vi "User Console View.vi"(8 "error in (no error)":errorcluster, 11 "View Model":T1) -> (0 "error out":errorcluster)   [LabVIEW 2017]
doc: "This simulated HW Console View. Contains human input."
uses:
  View Model/Controls/View Model.ctl
  Configuration/Controls/Config Model.ctl
  Configuration/Controls/Config Data.ctl
  Error Handler/Controls/Error Model.ctl
  Error Handler/Controls/Error Data.ctl
  Error Handler/Controls/Error Type.ctl
  View Model/Controls/Shared Model.ctl
  Elevator Controller/Controls/Elevator Model.ctl
  Elevator Controller/Controls/Elevator Location.ctl
  Elevator Controller/Controls/Elevator CMD Data.ctl
  Elevator Controller/Controls/Elevator Commands.ctl
  Elevator Controller/Controls/Elevator Overhead.ctl
  Elevator Controller/Controls/Elevator States.ctl
  Controls/User Console.ctl
panel:
  in  "Emergency":bool
  in  "1st Floor":bool
  in  "2nd Floor":bool
  in  "3rd Floor":bool
  in  "4th Floor":bool
  in  "Close Door":bool
  in  "Open Door":bool
  in  "Down 4":bool
  in  "Down 3":bool
  in  "Down 2":bool
  in  "Up 3":bool
  in  "Up 2":bool
  in  "Up 1":bool
  # "[Covers: UI1]"
  # "Floor Selection"
  # "Elevator Call"
  # "[Covers: UI2B]"
  # "[Covers UI2A1]"
  # "[Covers UI2A2]"
  # "[Covers UI2B2]"
  # "by controls mechanical actions"
  # "[Covers: UI2C]"
  # "[Covers: UI2D]"
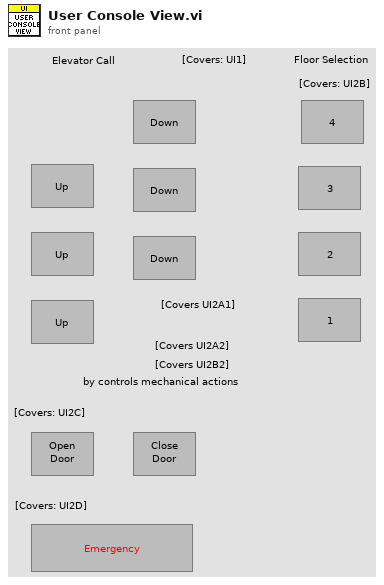
[diagram p1: front panel]
types:
  T1 = typedef "View Model.ctl" = cluster{"Config Model":T2, "Error Model":T3, "Shared Model":T4, "Elevator Model":T5}
  T2 = typedef "Config Model.ctl" = cluster{"Config Change":refnum<user-event>, "Config Data":refnum<data-value>}
  T3 = typedef "Error Model.ctl" = cluster{"Error Event":refnum<user-event>}
  T4 = typedef "Shared Model.ctl" = cluster{"Stop Event":refnum<user-event>, "Stop DVR":refnum<data-value>}
  T5 = typedef "Elevator Model.ctl" = cluster{"Motion Change":refnum<user-event>, "Direction Change":refnum<user-event>, "Door Position Change":refnum<user-event>, "Emergency Change":refnum<user-event>, "Floor Change":refnum<user-event>, "Elevator CMD":refnum<user-event>, "Controller Overhead":refnum<data-value>}
  T6 = typedef "User Console.ctl" = cluster{"Down 2":refnum<vi>, "Down 3":refnum<vi>, "Down 4":refnum<vi>, "Up 1":refnum<vi>, "Up 2":refnum<vi>, "Up 3":refnum<vi>, "1st Floor":refnum<vi>, "2nd Floor":refnum<vi>, "3rd Floor":refnum<vi>, "4th Floor":refnum<vi>, "Open Door":refnum<vi>, "Close Door":refnum<vi>, "Emergency":refnum<vi>}
  T7 = typedef "Elevator Commands.ctl" = enum16{"Go Up", "Go Down", "Go to Floor", "Emergency", "Open Doors", "Close Doors"}
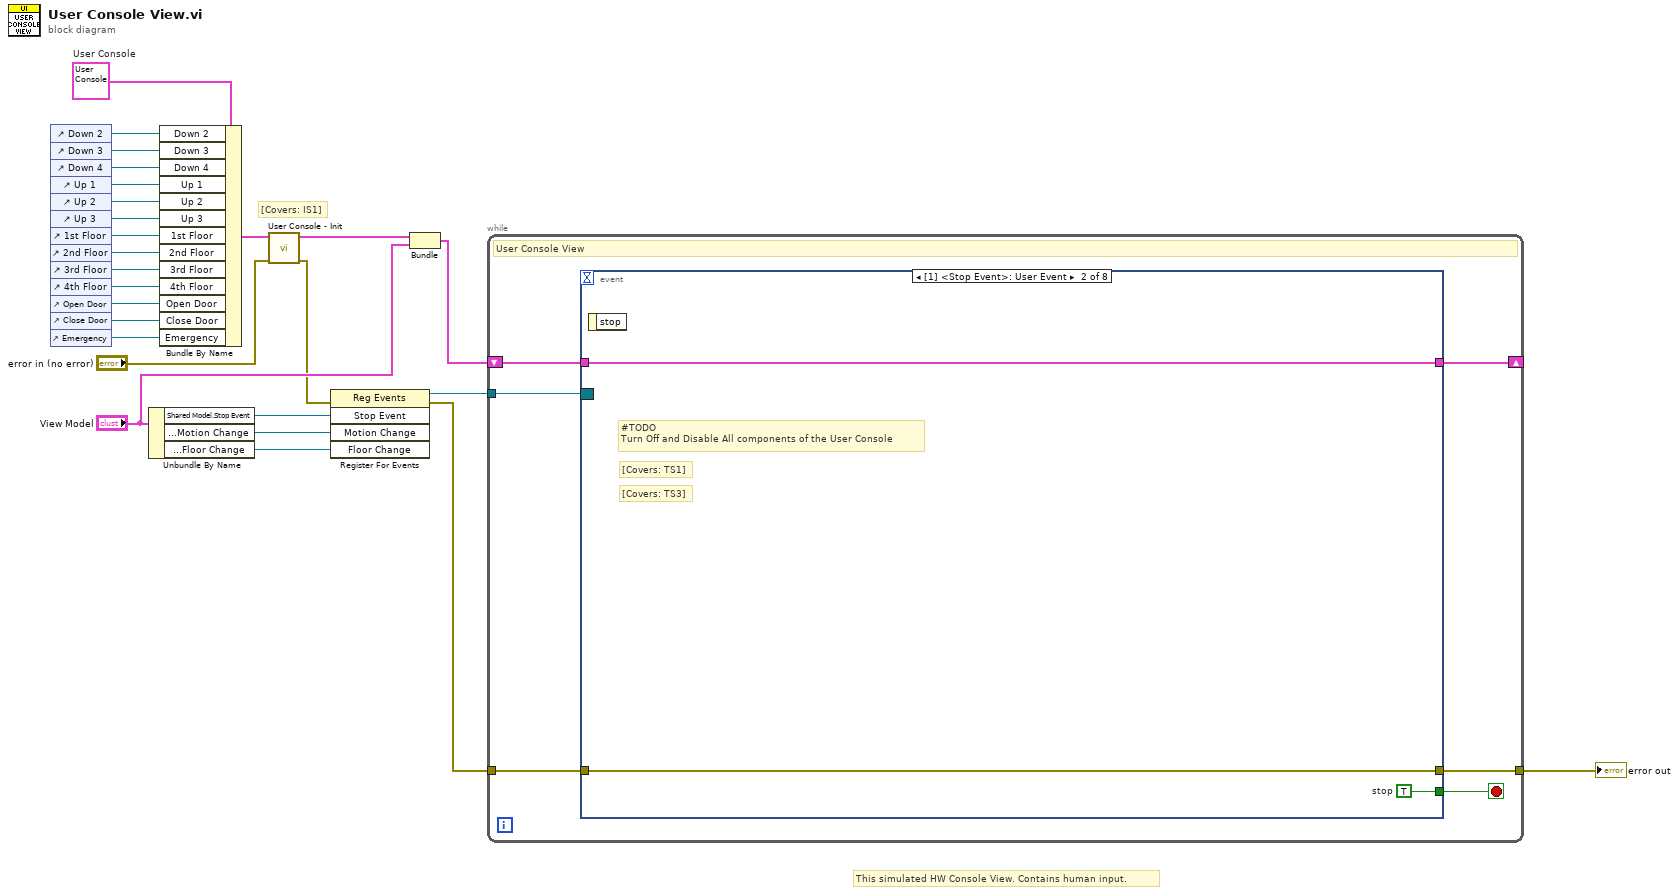
[diagram p0: block diagram]
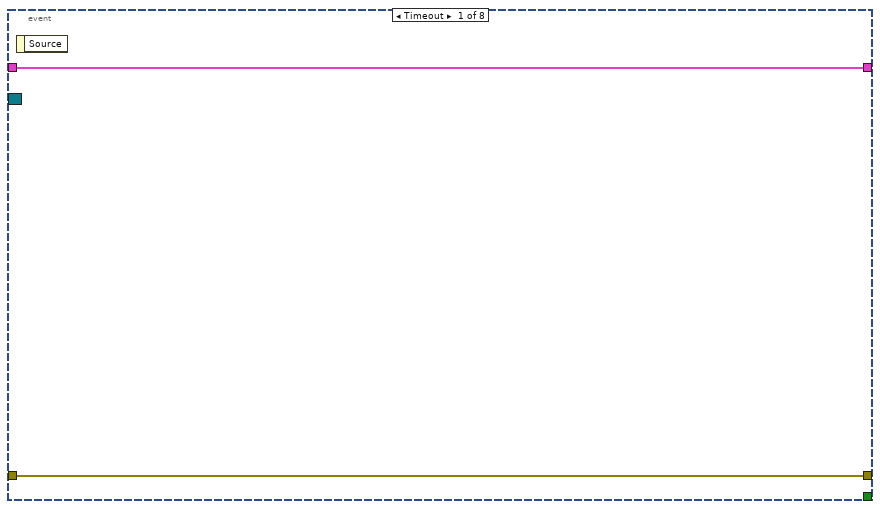
[diagram p2: hidden frame]
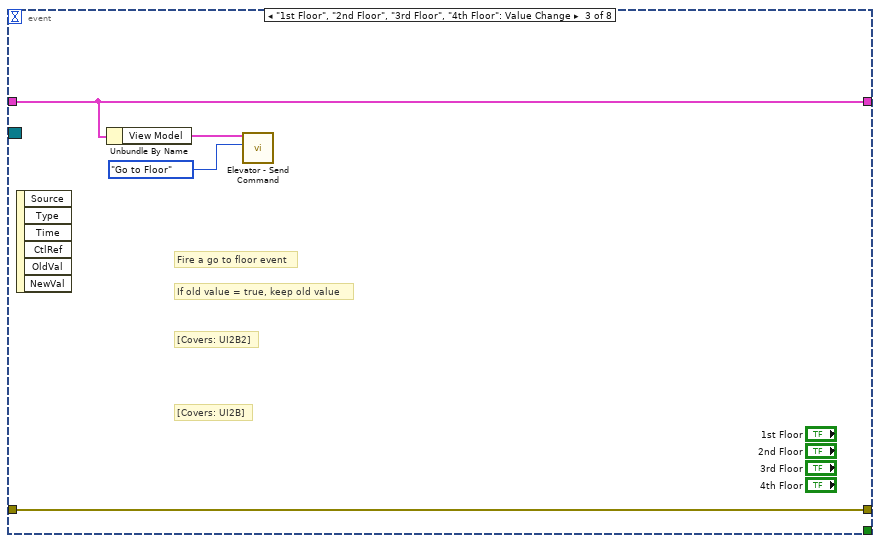
[diagram p3: hidden frame]
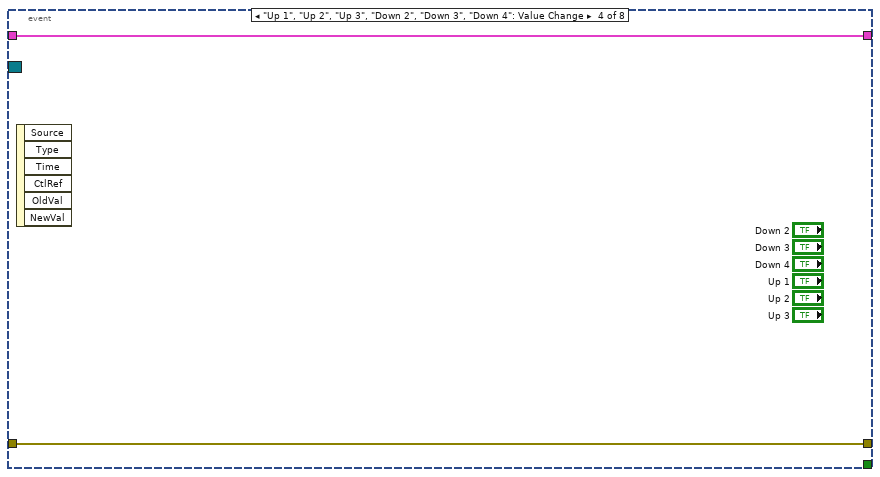
[diagram p4: hidden frame]
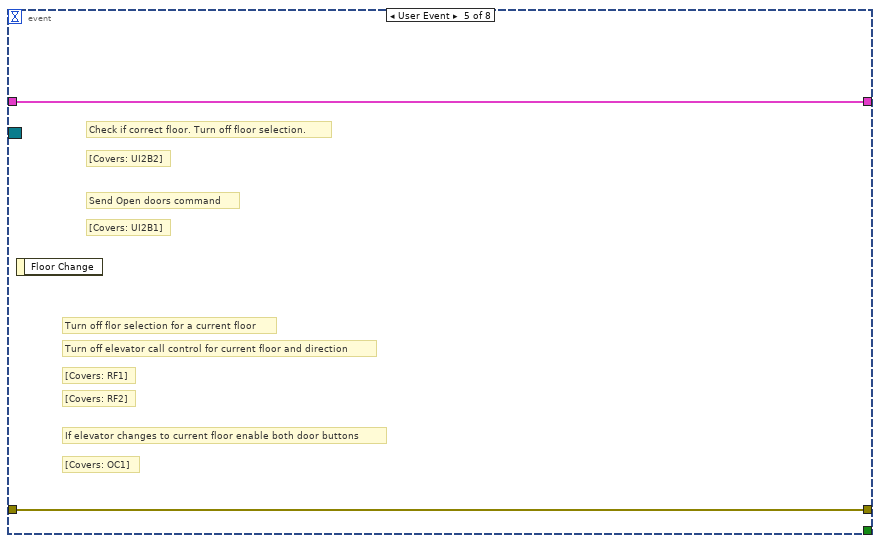
[diagram p5: hidden frame]
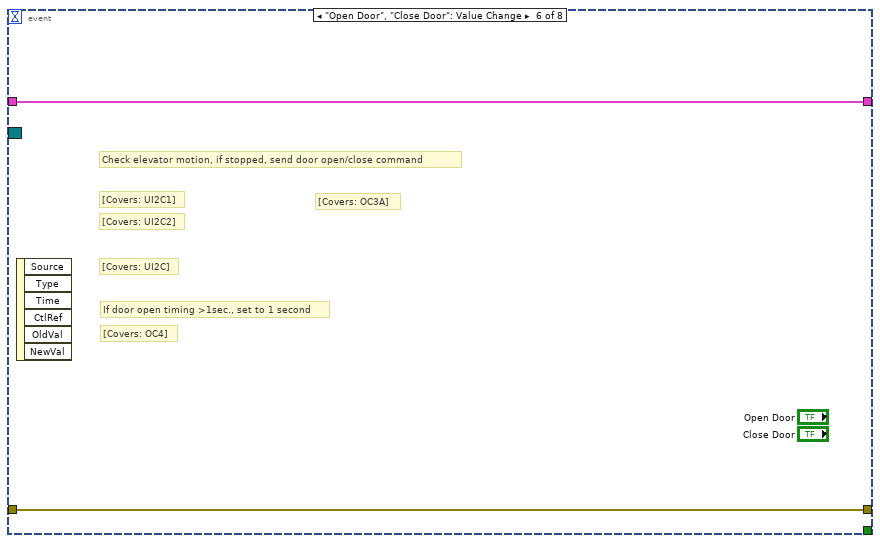
[diagram p6: hidden frame]
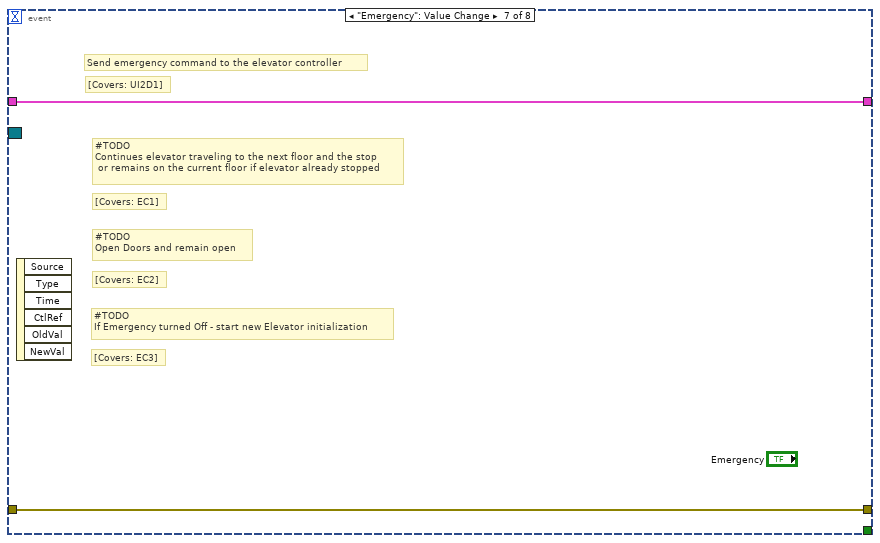
[diagram p7: hidden frame]
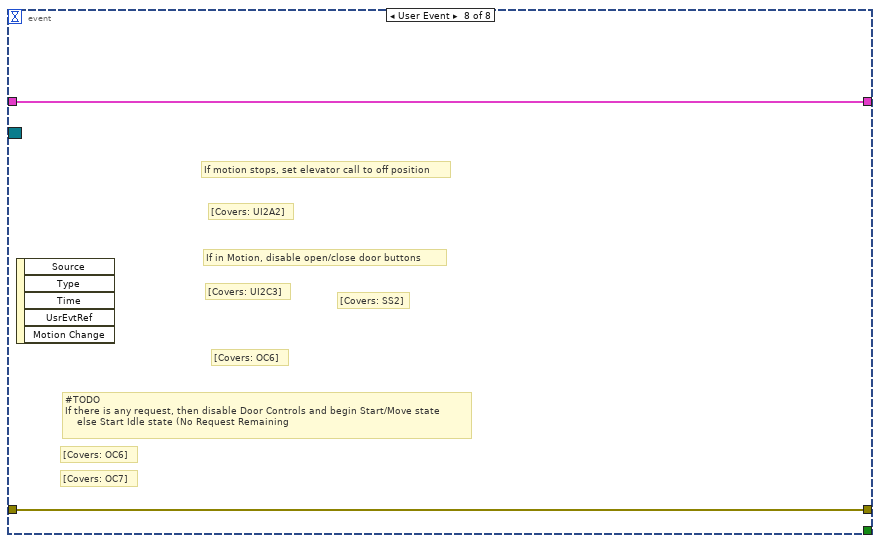
[diagram p8: hidden frame]
diagram:
  w22 = T6 {"Down 2"=refnum, "Down 3"=refnum, "Down 4"=refnum, "Up 1"=refnum, "Up 2"=refnum, "Up 3"=refnum, "1st Floor"=refnum, "2nd Floor"=refnum, "3rd Floor"=refnum, "4th Floor"=refnum, "Open Door"=refnum, "Close Door"=refnum, "Emergency"=refnum}  # User Console
  # "[Covers: IS1]"
  # "This simulated HW Console View. Contains human input."
  n1 = control-ref of="Down 2"() -> (w21:refnum<vi>)
  n2 = control-ref of="Down 3"() -> (w19:refnum<vi>)
  n3 = control-ref of="Down 4"() -> (w18:refnum<vi>)
  n4 = control-ref of="Up 1"() -> (w17:refnum<vi>)
  n5 = control-ref of="Up 2"() -> (w16:refnum<vi>)
  n6 = control-ref of="Up 3"() -> (w15:refnum<vi>)
  n7 = control-ref of="1st Floor"() -> (w14:refnum<vi>)
  n8 = control-ref of="2nd Floor"() -> (w13:refnum<vi>)
  n9 = control-ref of="3rd Floor"() -> (w12:refnum<vi>)
  n10 = control-ref of="4th Floor"() -> (w11:refnum<vi>)
  n11 = control-ref of="Open Door"() -> (w10:refnum<vi>)
  n12 = control-ref of="Close Door"() -> (w9:refnum<vi>)
  n13 = control-ref of="Emergency"() -> (w20:refnum<vi>)
  n14 = Unbundle By Name("View Model") -> ("Shared Model.Stop Event"=w26:refnum<user-event>, "Elevator Model.Motion Change"=w25:refnum<user-event>, "Elevator Model.Floor Change"=w1:refnum<user-event>)
  n15 = Bundle By Name(cluster=w22, "Down 2"=w21, "Down 3"=w19, "Down 4"=w18, "Up 1"=w17, "Up 2"=w16, "Up 3"=w15, "1st Floor"=w14, "2nd Floor"=w13, "3rd Floor"=w12, "4th Floor"=w11, "Open Door"=w10, "Close Door"=w9, "Emergency"=w20) -> (w8:T6)
  n16 = call "User Console - Init.vi"("error in (no error)"="error in (no error)", "User Console"=w8) -> ("error out"=w4:errorcluster, "User Console"=w7:T6)  [unwired: 8 in]
  n17 = register-events(error in=w4, w26, w25, w1) -> (reference out=w24:refnum<event-registration>, error out=w3:errorcluster)  [unwired: 1 in]
  n18 = Bundle("User Console"=w7, "View Model"="View Model") -> (w2:cluster{"User Console":T6, "View Model":T1})  [unwired: 1 in]
  n19 = while {
    tunnel: w24 -> [w32]
    tunnel: w3 -> [w31]
    tunnel: [w30] -> w23
    shift-right: [w27] -> _
    shift-left: w2 -> [w28]
    stop <- w29 stop-if-true
    # "User Console View"
    n20 = event shown="[1] <Stop Event>: User Event" {
      selector: w32 -> [_ _ _ _ _ _ _ _]
      dyn-events: _ -> [_ _ _ _ _ _ _ _]
      timeout: _ -> [_ _ _ _ _ _ _ _]
      tunnel: w31 -> [w34 w35 w41 w43 w45 w47 w49 w51]
      tunnel: [w34 w35 w41 w43 w45 w47 w49 w51] -> w30
      tunnel: [_ w37 _ _ _ _ _ _] -> w29
      tunnel: w28 -> [w33 w36 w40 w42 w44 w46 w48 w50]
      tunnel: [w33 w36 w40 w42 w44 w46 w48 w50] -> w27
      event Timeout {
        n21 = event-data() -> ()  [unwired: 1 in, 1 out]
      }
      event User Event {
        w37 = TRUE  # stop
        # "[Covers: TS3]"
        # "[Covers: TS1]"
        # "#TODO\nTurn Off and Disable All components of the User Console"
        n22 = event-data() -> ()  [unwired: 1 in, 1 out]
      }
      event "1st Floor", "2nd Floor", "3rd Floor", "4th Floor": Value Change {
        # "[Covers: UI2B]"
        # "[Covers: UI2B2]"
        # "If old value = true, keep old value"
        # "Fire a go to floor event"
        n23 = event-data() -> ()  [unwired: 1 in, 6 out]
        n24 = Unbundle By Name(w40) -> ("View Model"=w39:T1)
        n25 = call "Elevator - Send Command.vi"("Elevator Commands"=Elevator_Commands."Go to Floor", "View Model"=w39) -> ()  [unwired: 8 in, 2 out]
      }
      event "Up 1", "Up 2", "Up 3", "Down 2", "Down 3", "Down 4": Value Change {
        n26 = event-data() -> ()  [unwired: 1 in, 6 out]
      }
      event User Event {
        # "[Covers: UI2B1]"
        # "Send Open doors command"
        # "Check if correct floor. Turn off floor selection."
        # "[Covers: UI2B2]"
        # "[Covers: OC1]"
        # "If elevator changes to current floor enable both door buttons"
        # "[Covers: RF2]"
        # "Turn off elevator call control for current floor and direction"
        # "[Covers: RF1]"
        # "Turn off flor selection for a current floor"
        n27 = event-data() -> ()  [unwired: 1 in, 1 out]
      }
      event "Open Door", "Close Door": Value Change {
        # "[Covers: OC3A]"
        # "[Covers: UI2C]"
        # "[Covers: UI2C2]"
        # "[Covers: UI2C1]"
        # "Check elevator motion, if stopped, send door open/close command"
        # "[Covers: OC4]"
        # "If door open timing >1sec., set to 1 second"
        n28 = event-data() -> ()  [unwired: 1 in, 6 out]
      }
      event "Emergency": Value Change {
        # "[Covers: EC3]"
        # "#TODO\nIf Emergency turned Off - start new Elevator initialization"
        # "[Covers: EC2]"
        # "[Covers: EC1]"
        # "#TODO\nOpen Doors and remain open"
        # "#TODO\nContinues elevator traveling to the next floor and the stop\n or remains on the current floor if elevator already stopped"
        # "[Covers: UI2D1]"
        # "Send emergency command to the elevator controller"
        n29 = event-data() -> ()  [unwired: 1 in, 6 out]
      }
      event User Event {
        # "[Covers: OC7]"
        # "[Covers: OC6]"
        # "#TODO\nIf there is any request, then disable Door Controls and begin Start/Move state\n    else Start Idle state (No Request Remaining"
        # "[Covers: OC6]"
        # "[Covers: SS2]"
        # "[Covers: UI2C3]"
        # "If in Motion, disable open/close door buttons"
        # "[Covers: UI2A2]"
        # "If motion stops, set elevator call to off position"
        n30 = event-data() -> ()  [unwired: 1 in, 5 out]
      }
    }
  }
  "error out" <- w23
